vi "Set Fast Run Parameters.vi"(8 "Error in":errorcluster caption="错误输入", 9 "Full Speed Config":T1={"Drive Force"=80, "Run Speed"=300, "Speed Unit"="rpm", "Full Drive Force Unit"=0} caption="全速运行参数" {"Full Drive Force Unit" items=["%"]; "Run Speed" min=100 max=300 step=1; "Drive Force" min=20 max=100 step=1}, 10 "Channel":dbl=1.0 caption="设备通道", 11 "Modbus instance in":refnum<class "Modbus API.lvclass"> caption="Modbus实例输入") -> (0 "Error out":errorcluster caption="错误输出", 3 "Modbus instance out":refnum<class "Modbus API.lvclass"> caption="Modbus实例输出")   [LabVIEW 2023, in "Longer Pump dLSP501 Series.lvlib"]
uses:
  <instrlib>/Longer Pump dLSP501 Modbus RTU Series/Longer Pump dLSP501 Series.lvlib
  <vilib>/NI/Modbus Library/API/Modbus API.lvclass
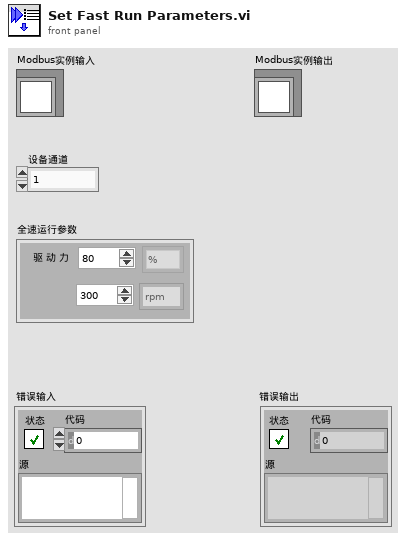
[diagram p1: front panel]
types:
  T1 = cluster{"Drive Force":u16, "Run Speed":u16, "Speed Unit":string, "Full Drive Force Unit":u16}
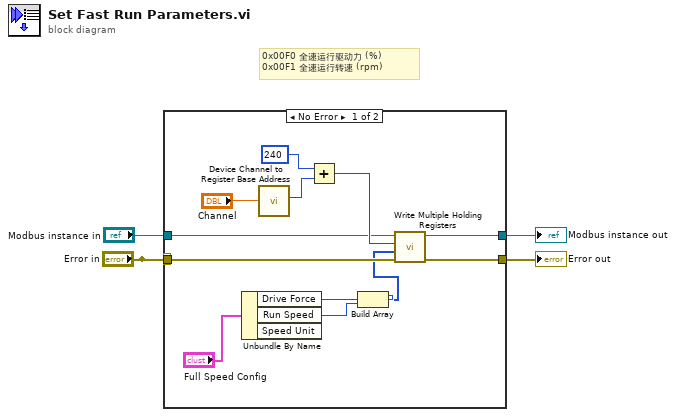
[diagram p0: block diagram]
diagram:
  # "0x00F0\t全速运行驱动力 (%)\n0x00F1\t全速运行转速 (rpm)"
  n1 = case shown="No Error" "Error in" {
    selector: "Error in" -> [_ w17]
    tunnel: "Error in" -> [w16 _]
    tunnel: "Modbus instance in" -> [w9 w18]
    tunnel: [w15 w17] -> w1
    tunnel: [w14 w18] -> w3
    frame No Error {
      n2 = Unbundle By Name("Full Speed Config") -> ("Drive Force"=w7:u16, "Run Speed"=w6:u16)  [unwired: 1 out]
      n3 = call <instrlib>:"Device Channel to Register Base Address.vi"("Channel"="Channel") -> ("Register Base Address"=w12:u16)  [unwired: 10 in]
      n4 = Add(x=u16 240 ("address"), y=w12) -> (x+y=w10:u16)
      n5 = Build Array(w7, w6) -> (w5:u16[])
      n6 = call-dynamic "Write Multiple Holding Registers.vi"("error in"=w16, "registers to write"=w5, "starting address"=w10, "Modbus instance in"=w9) -> ("error out"=w15:errorcluster, "Modbus instance out"=w14:refnum<class "Modbus API.lvclass">)  [unwired: 6 in]
    }
    frame Error {
    }
  }
  "Modbus instance out" <- w3
  "Error out" <- w1
